vi "take_screenshot.vi"(5 "String in":refnum<vi>, 6 "Visible area only? (f)":bool, 7 "error in (no error)":errorcluster, 8 "Enum in":refnum<vi>, 10 "VI in":refnum<vi>) -> (0 "error out":errorcluster, 2 "Image path":path)   [LabVIEW 2018]
doc: "This example captures an image of the front panel of a VI and saves the image to a JPG, PNG, or BMP file."
panel:
  out "Base64 String":string
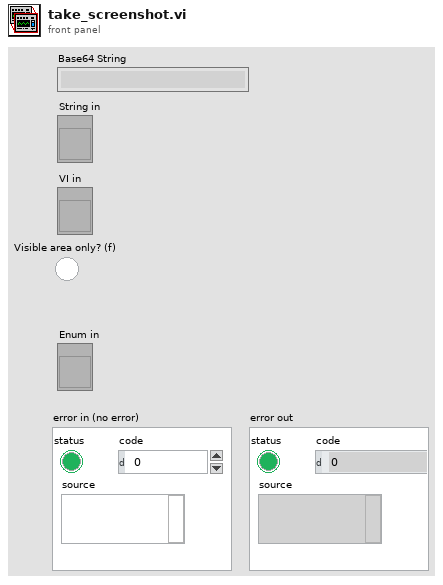
[diagram p1: front panel]
types:
  T1 = typedef "imagedata.ctl" = cluster{"image type":i32, "image depth":i32, "image":u8[], "mask":u8[], "colors":u32[], "Rectangle":cluster{"left":i16, "top":i16, "right":i16, "bottom":i16}}
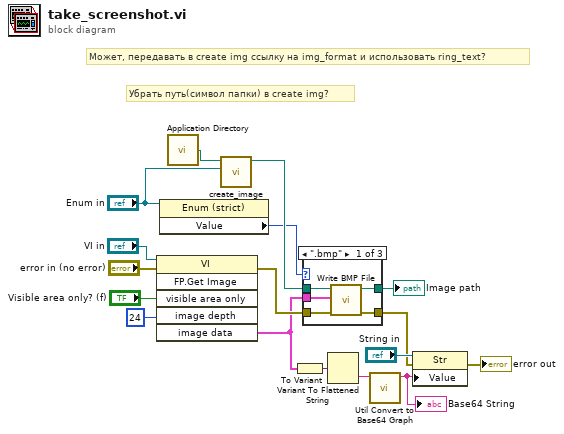
[diagram p0: block diagram]
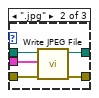
[diagram p2: hidden frame]
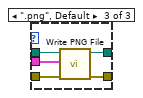
[diagram p3: hidden frame]
diagram:
  # "Убрать путь(символ папки) в create img?"
  # "Может, передавать в create img ссылку на img_format и использовать ring_text?"
  n1 = invoke class="VI" method="FP.Get Image"(reference="VI in", error in="error in (no error)", "visible area only"="Visible area only? (f)", "image depth"=24 ("Image Depth")) -> (error out=w17:errorcluster, "image data"=w7:T1)  [unwired: 2 in, 4 out]
  n2 = property class="Enum (strict)"(reference="Enum in") -> ("Value"=w1:enum32{".png", ".jpg", ".bmp"})  [unwired: 1 in, 2 out]
  n3 = call <vilib>:"Application Directory.vi"() -> ("Application Directory"=w4:path)
  n4 = call "create_image.vi"("Enum in"="Enum in", "base path"=w4) -> ("path"=w3:path)  [unwired: 8 in, 1 out]
  n5 = To Variant(anything=w7) -> (Variant=w9:variant)
  n6 = case shown="\".bmp\"" w1 {
    tunnel: w7 -> [w21 w26 w31]
    tunnel: w17 -> [w20 w27 w32]
    tunnel: w3 -> [w22 w25 w30]
    tunnel: [w19 w24 w29] -> w6
    tunnel: [w18 w23 w28] -> w15
    frame ".bmp" {
      n7 = call <vilib>:"Write BMP File.vi"("error in (no error)"=w20, "image data"=w21, "path to BMP file"=w22) -> ("error out"=w19:errorcluster, "path"=w18:path)  [unwired: 7 in]
    }
    frame ".jpg" {
      n8 = call <vilib>:"Write JPEG File.vi"("error in (no error)"=w27, "image data"=w26, "path to JPEG file"=w25) -> ("error out"=w24:errorcluster, "path"=w23:path)  [unwired: 7 in]
    }
    frame ".png", Default {
      n9 = call <vilib>:"Write PNG File.vi"("error in (no error)"=w32, "image data"=w31, "path to PNG file"=w30) -> ("error out"=w29:errorcluster, "path"=w28:path)  [unwired: 7 in]
    }
  }
  "Image path" <- w15
  n10 = Variant To Flattened String(Variant=w9) -> (data string=w10:string)  [unwired: 1 out]
  n11 = call "Util Convert to Base64 Graph.vi"("String"=w10) -> ("Base64 String"=w11:string)  [unwired: 10 in]
  "Base64 String" <- w11
  n12 = property on="Property Node" class="Str"(reference="String in", error in=w6, "Value"=w11) -> (error out=→"error out":errorcluster)  [unwired: 1 out]
